vi "SwissSPAD Live_Download Multiple Images_v4.vi"(6 "Block Size (-1-> 16,384)":i32=-1, 8 "Error In":errorcluster, 9 "# 8-bit Images (1)":u32=1, 10 "Buffer Size (# 8-bit Images)":u32, 11 "SwissSPAD Live Internal Variables":T1={"okCFrontPanelDevices Refnum"=refnum, "Bottom Device Refnum"=refnum, "Display Image"=refnum, "# Live Images"=0, "relative s"=0.0, "# Image Sets"=0, "Message"="", "Current Image Set"=0, "# Datasets in Series"=0, "Current Dataset"=0, "Live Mode"=FALSE, "Recording Mode"=FALSE, "Record Button"=refnum, "\nLive Button"=refnum, "SwissSPAD Live Gate Image Data Q Name"="SS2 Live Gate Data Q", "Discard First Image"=FALSE, "Image Information"={"Save ROI Only"=FALSE, "Left"=0, "Top"=0, "Right"=0, "Bottom"=0, "Use Current ROI"=FALSE}, "Image Binning Options"={"Use Image Binning"=FALSE, "X Bin"=1, "Y Bin"=1}, "Bottom FPGA Serial Number"="", "Detector PCB Version"=enum."SS2 PCB1", "# Acquisitions"=1, "10 bits"=FALSE, "Top FPGA Serial Number"="", "Top Device Refnum"=refnum} {"# Acquisitions" min=1; "Image Binning Options"."Y Bin" min=1; "Image Binning Options"."X Bin" min=1}) -> (0 "Error Out":errorcluster, 3 "SwissSPAD Live Internal Variables":T1={"okCFrontPanelDevices Refnum"=refnum, "Bottom Device Refnum"=refnum, "Display Image"=refnum, "# Live Images"=0, "relative s"=0.0, "# Image Sets"=0, "Message"="", "Current Image Set"=0, "# Datasets in Series"=0, "Current Dataset"=0, "Live Mode"=FALSE, "Recording Mode"=FALSE, "Record Button"=refnum, "\nLive Button"=refnum, "SwissSPAD Live Gate Image Data Q Name"="SS2 Live Gate Data Q", "Discard First Image"=FALSE, "Image Information"={"Save ROI Only"=FALSE, "Left"=0, "Top"=0, "Right"=0, "Bottom"=0, "Use Current ROI"=FALSE}, "Image Binning Options"={"Use Image Binning"=FALSE, "X Bin"=1, "Y Bin"=1}, "Bottom FPGA Serial Number"="", "Detector PCB Version"=enum."SS2 PCB1", "# Acquisitions"=1, "10 bits"=FALSE, "Top FPGA Serial Number"="", "Top Device Refnum"=refnum} {"# Acquisitions" min=1; "Image Binning Options"."Y Bin" min=1; "Image Binning Options"."X Bin" min=1})   [LabVIEW 2021]
uses:
  SwissSPAD Live_Internal Variables.ctl
  D:/UCLA Thinkpad Google Drive/LabVIEW 2021 SP1/builds/SwissSPAD Live Distribution/Opal Kelly/C# Wrapper/v5.0.2/libFrontPanel-csharp.dll
  Opal Kelly/C# Wrapper/v5.0.2/libFrontPanel-csharp.dll
  <vilib>/vision/Image Controls.llb/IMAQ Image.ctl
  SwissSPAD Live_Image ROI Information.ctl
  Phasor/Image Binning Options.ctl
  SwissSPAD Live_SSx PCB Version.ctl
  <vilib>/Utility/error.llb/Error Cluster From Error Code.vi
  <vilib>/ErrorRing/Error Ring.xnode
  Opal Kelly/C# Wrapper/okFrontPanelC#Wrapper.lvlib
  Notebook/Notebook.lvlib
  Rich Text Box/Rich Text Box.lvlib
panel:
  out "Last Iteration Index":i32
  out "Enqueue error out":errorcluster
  out "# Buffers reads":i32
  out "Bytes Transferred":i32
  out "ReadFromBlockPipeout Error":errorcluster
  out "Activate Trigger Error Out":errorcluster
  out "Timeout error":errorcluster
  out "CPU/8-bit Gate":dbl
  in  "Discard First Image":bool
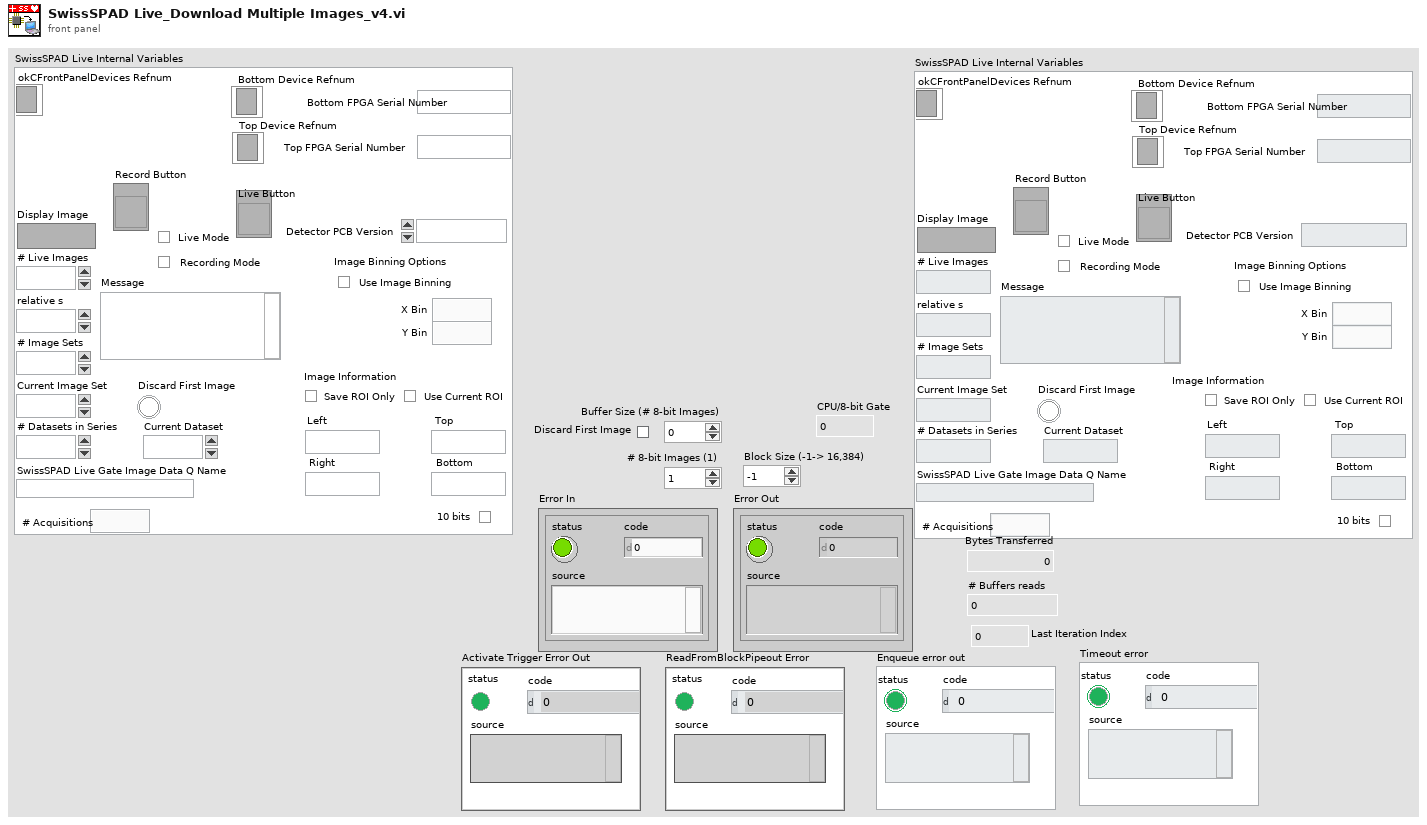
[diagram p1: front panel]
types:
  T1 = typedef "SwissSPAD Live_Internal Variables.ctl" = cluster{"okCFrontPanelDevices Refnum":refnum<k24>, "Bottom Device Refnum":refnum<k24>, "Display Image":T2, "# Live Images":i32, "relative s":dbl, "# Image Sets":i32, "Message":string, "Current Image Set":i32, "# Datasets in Series":i32, "Current Dataset":i32, "Live Mode":bool, "Recording Mode":bool, "Record Button":refnum<vi>, "\nLive Button":refnum<vi>, "SwissSPAD Live Gate Image Data Q Name":string, "Discard First Image":bool, "Image Information":T3, "Image Binning Options":T4, "Bottom FPGA Serial Number":string, "Detector PCB Version":T5, "# Acquisitions":u32, "10 bits":bool, "Top FPGA Serial Number":string, "Top Device Refnum":refnum<k24>}
  T2 = typedef "IMAQ Image.ctl" = refnum<image>
  T3 = typedef "SwissSPAD Live_Image ROI Information.ctl" = cluster{"Save ROI Only":bool, "Left":u16, "Top":u16, "Right":u16, "Bottom":u16, "Use Current ROI":bool}
  T4 = typedef "Image Binning Options.ctl" = cluster{"Use Image Binning":bool, "X Bin":i32, "Y Bin":i32}
  T5 = typedef "SwissSPAD Live_SSx PCB Version.ctl" = enum16{"unknown", "SS2 PCB1", "SS2 PCB2", "SS3 PCB1"}
  T6 = typedef "Rich Text Box.lvlib/Text Formatting.ctl" = cluster{"Font":string, "Text Color":T7, "Text Background Color":T7, "Text Style":enum16{"Regular", "Bold", "Italic", "Underline", "Strikeout"}, "Font Size (Points)":dbl, "Text Alignment":i32}
  T7 = typedef "Rich Text Box.lvlib/Text Colors.ctl" = enum16{"Unchanged", "Black", "Blue", "Brown", "Gray", "Green", "Orange", "Pink", "Red", "White"}
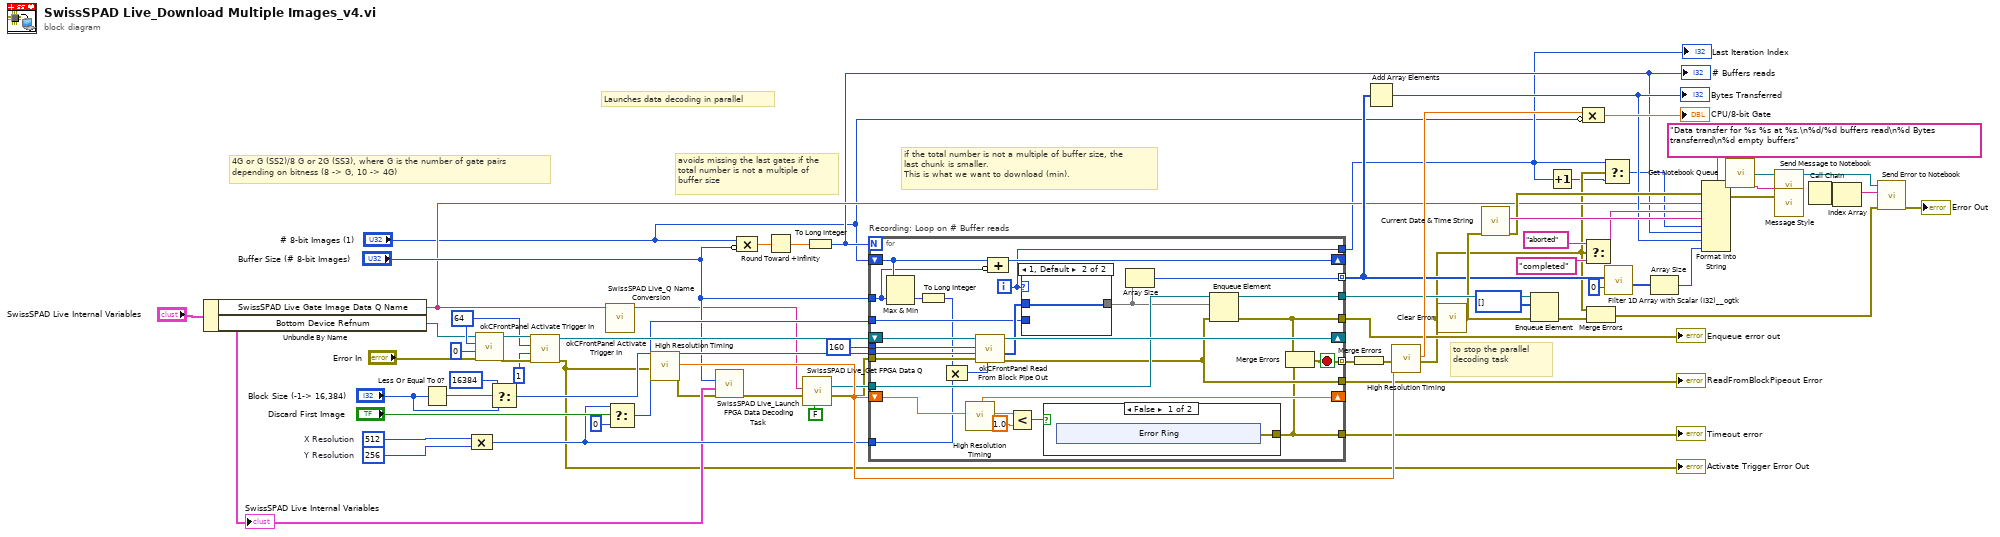
[diagram p0: block diagram]
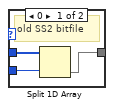
[diagram p3: hidden frame]
diagram:
  w38 = 256  # Y Resolution
  w62 = 512  # X Resolution
  w67 = 64 ("Endpoint Addr")
  # "to stop the parallel decoding task"
  # "Launches data decoding in parallel"
  # "if the total number is not a multiple of buffer size, the last chunk is smaller.\nThis is what we want to download (min)."
  # "avoids missing the last gates if the total number is not a multiple of buffer size"
  # "4G or G (SS2)/8 G or 2G (SS3), where G is the number of gate pairs\ndepending on bitness (8 -> G, 10 -> 4G)"
  n1 = Unbundle By Name("SwissSPAD Live Internal Variables") -> ("SwissSPAD Live Gate Image Data Q Name"=w11:string, "Bottom Device Refnum"=w37:refnum<k24>)
  n2 = Less Or Equal To 0?(x="Block Size (-1-> 16,384)") -> (x <= 0?=w65:bool)
  n3 = Compound Arithmetic op=MULTIPLY(w62, w38) -> (w33:i32)
  n4 = call "okCFrontPanel Activate Trigger In.vi"("Error In"="Error In", "Bit"=0, "Endpoint Addr"=w67, "okCFrontPanel Refnum"=w37) -> ("Error Out"=w69:errorcluster, "okCFrontPanel Refnum"=w68:refnum<k24>)  [unwired: 6 in]
  n5 = Select(t=16384, s=w65, f="Block Size (-1-> 16,384)") -> (s? t:f=w55:i32)
  n6 = call "okCFrontPanel Activate Trigger In.vi"("Error In"=w69, "Bit"=1, "Endpoint Addr"=w67, "okCFrontPanel Refnum"=w68) -> ("Error Out"=w22:errorcluster, "okCFrontPanel Refnum"=w56:refnum<k24>)  [unwired: 6 in]
  "Activate Trigger Error Out" <- w22
  n7 = call "SwissSPAD Live_Q Name Conversion.vi"("SwissSPAD Live Gate Data Decode Q Name"=w11) -> ("FPGA Q Name"=w10:string)  [unwired: 10 in]
  n8 = Select(t=w33, s="Discard First Image", f=0) -> (s? t:f=w54:i32)
  n9 = call "High Resolution Timing.vi"("Error In"=w22) -> ("elapsed (relative) seconds"=w48:dbl, "Error Out"=w27:errorcluster)  [unwired: 16 in, 1 out]
  n10 = call "SwissSPAD Live_Launch FPGA Data Decoding Task.vi"("error in (no error)"=w27, "SwissSPAD Live Internal Variables"="SwissSPAD Live Internal Variables", "Buffer Size (# 8-bit images)"="Buffer Size (# 8-bit Images)") -> ("error out"=w16:errorcluster)  [unwired: 8 in]
  n11 = Compound Arithmetic op=MULTIPLY("# 8-bit Images (1)", invert "Buffer Size (# 8-bit Images)") -> (w42:dbl)
  n12 = Round Toward +Infinity(x=w42) -> (ceil(x): smallest int >= x=w43:dbl)
  n13 = call "SwissSPAD Live_Get FPGA Data Q.vi"("create if not found? (T)"=FALSE, "error in (no error)"=w16, "FPGA Data Q Name"=w10) -> ("error out"=w18:errorcluster, "FPGA Data Q"=w19:refnum<queue>)  [unwired: 7 in]
  n14 = To Long Integer(number=w43) -> (32bit integer=w7:i32)
  "# Buffers reads" <- w7
  n15 = for "Recording: Loop on # Buffer reads" {
    N: w7 -> [_]
    tunnel: 160 ("Endpoint Addr") -> [w97]
    shift-right: [w95] -> _
    shift-left: w56 -> [w96]
    tunnel: w55 -> [w93]
    tunnel: w54 -> [w86]
    tunnel: w19 -> [w92]
    tunnel: [w79] -> w52 mode=indexing
    tunnel: [w91] -> w49
    shift-right: [w87] -> _
    shift-left: w48 -> [w90]
    shift-right: [w85] -> _
    shift-left: "# 8-bit Images (1)" -> [w84]
    tunnel: "Buffer Size (# 8-bit Images)" -> [w83]
    tunnel: w33 -> [w81]
    tunnel: w18 -> [w78]
    tunnel: [w76] -> w15 mode=indexing
    tunnel: [w75] -> w24
    tunnel: [w73] -> w23
    tunnel: [w72] -> w25
    tunnel: [w71] -> w4
    i -> [w71]
    stop <- w79 stop-if-true
    n16 = Max & Min(x=w84, y=w83) -> (min(x,y)=w82:u32)  [unwired: 1 out]
    n17 = To Long Integer(number=w82) -> (32bit integer=w70:i32)
    n18 = Compound Arithmetic op=MULTIPLY(w70, w81) -> (w80:i32)
    n19 = call "High Resolution Timing.vi"("relative seconds (NaN)"=w90) -> ("relative seconds"=w87:dbl, "elapsed (relative) seconds"=w89:dbl)  [unwired: 16 in, 1 out]
    n20 = call "okCFrontPanel Read From Block Pipe Out.vi"("Length"=w80, "Error In"=w78, "Block Size"=w93, "Endpoint Addr"=w97, "okCFrontPanel Refnum"=w96) -> ("Error Out"=w75:errorcluster, "BYTEARRAY"=w94:u8[], "okCFrontPanel Refnum"=w95:refnum<k24>)  [unwired: 4 in]
    n21 = Compound Arithmetic op=ADD(w84, invert w83) -> (w85:u32)
    n22 = Less?(x=w89, y=1.0) -> (x < y?=w74:bool)
    n23 = case shown="1, Default" w71 {
      tunnel: w94 -> [w105 w106]
      tunnel: w86 -> [w104 _]
      tunnel: [w103 w106] -> w77
      frame 0 {
        # "old SS2 bitfile"
        n24 = Split 1D Array(array=w105, index=w104) -> (second subarray=w103:u8[])  [unwired: 1 out]
      }
      frame 1, Default {
      }
    }
    n25 = case shown="False" w74 {
      tunnel: [w98 _] -> w73
      frame False {
        n26 = xnode "Error Ring"() -> ("error out"=w98:errorcluster)
      }
      frame True {
      }
    }
    n27 = Array Size(array=w77) -> (size(s)=w76:i32)
    n28 = Enqueue Element(queue=w92, element=w77, error in (no error)=w75) -> (queue out=w91:refnum<queue>, error out=w72:errorcluster)  [unwired: 1 in, 1 out]
    n29 = Merge Errors(w72, w73) -> (w79:errorcluster)
  }
  "Timeout error" <- w23
  "ReadFromBlockPipeout Error" <- w24
  "Enqueue error out" <- w25
  "Last Iteration Index" <- w4
  n30 = Merge Errors(w52) -> (w50:errorcluster)
  n31 = Add Array Elements(numeric array=w15) -> (sum=w28:i32)
  "Bytes Transferred" <- w28
  n32 = call "High Resolution Timing.vi"("relative seconds (NaN)"=w48, "Error In"=w50) -> ("elapsed (relative) seconds"=w51:dbl, "Error Out"=w6:errorcluster)  [unwired: 15 in, 1 out]
  n33 = call "Clear Error.vi"("Error In"=w6) -> ("no Error Out"=w32:errorcluster)  [unwired: 8 in]
  n34 = call "Current Date & Time String.vi"("Error In"=w32) -> ("Error Out"=w39:errorcluster, "time string"=w40:string)  [unwired: 8 in, 1 out]
  n35 = Enqueue Element(queue=w49, element=u8[] [], error in (no error)=w32) -> (error out=w31:errorcluster)  [unwired: 1 in, 2 out]
  n36 = Increment(x=w4) -> (x+1=w5:i32)
  n37 = Compound Arithmetic op=MULTIPLY(w51, invert "# 8-bit Images (1)") -> (→"CPU/8-bit Gate":dbl)
  n38 = Select(t="aborted" ("input 2"), s=w6, f="completed" ("input 2")) -> (s? t:f=w34:string)
  n39 = Merge Errors(w6, w31) -> (w9:errorcluster)
  n40 = Select(t=w4, s=w6, f=w5) -> (s? t:f=w3:i32)
  n41 = call <userlib>:"Filter 1D Array with Scalar (I32)__ogtk.vi"("items to filter"=0, "array"=w15) -> ("filtered item indices"=w13:i32[])  [unwired: 4 in, 1 out]
  n42 = Array Size(array=w13) -> (size(s)=w12:i32)
  n43 = Format Into String(format string="Data transfer for %s %s at %s.\n%d/%d buffers read\n%d Bytes transferred\n%d empty buffers", error in=w39, w11, w34, w40, w3, w7, w28, w12) -> (resulting string=w45:string, error out=w41:errorcluster)  [unwired: 1 in]
  n44 = call "Get Notebook Queue.vi"() -> ("Notebook Queue"=w26:refnum<queue>)  [unwired: 9 in]
  n45 = call "Message Style.vi"() -> ("Message Formatting"=w47:T6)
  n46 = call "Send Message to Notebook.vi"("Text Formatting"=w47, "Error In"=w41, "Message"=w45, "Notebook Queue"=w26) -> ("Notebook Queue"=w1:refnum<queue>)  [unwired: 4 in, 1 out]
  n47 = Call Chain() -> (call chain=w21:string[])
  n48 = Index Array(array=w21) -> (element=w20:string)  [unwired: 1 in]
  n49 = call "Send Error to Notebook.vi"("error in (no error)"=w9, "State Machine Case Error Source"=w20, "Notebook Q"=w1) -> ("Error Out"=→"Error Out":errorcluster)  [unwired: 8 in]
  "SwissSPAD Live Internal Variables" <- "SwissSPAD Live Internal Variables"
